vi "Read Box State.vi"(11 "Box in":refnum<class "Box.lvclass">) -> (2 "box state":T1)   [LabVIEW 2023, in "Box.lvclass"]
uses:
  Box.lvclass
  Box State.ctl
  Box.lvclass/Box.ctl
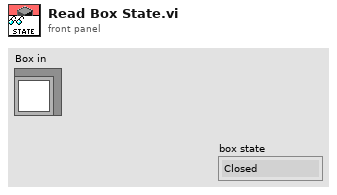
[diagram p1: front panel]
types:
  T1 = typedef "Box.lvclass/Box State.ctl" = enum16{"Closed", "Open"}
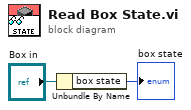
[diagram p0: block diagram]
diagram:
  n1 = Unbundle By Name("Box in") -> ("box state"=→"box state":T1)
